vi "get swerve refs.vi"(8 "error in (no error)":errorcluster) -> (0 "error out":errorcluster, 2 "Swerve refs":cluster{"Driver":T1, "Steer":T1, "Encoder":T6}[](array[cluster]))   [LabVIEW 2023]
uses:
  <vilib>/Rock Robotics/WPI/MotorControl/WPI_MotorControlDeviceRef.ctl
  <vilib>/Rock Robotics/WPI/MotorControl/WPI_MotorControlType.ctl
  <vilib>/Rock Robotics/SystemInterfaces/DIO/FPGA_DIOPWMChannel.ctl
  <vilib>/Rock Robotics/WPI/PWM/WPI_PWMDeadband.ctl
  <vilib>/Rock Robotics/SystemInterfaces/DIO/FPGA_DIOChannel.ctl
  <vilib>/Rock Robotics/WPI/ThirdParty/Phoenix-LabVIEW/CANCoder/Controls/CTRE_Phoenix_CANcoder_DeviceRef.ctl
  Global INIT.vi
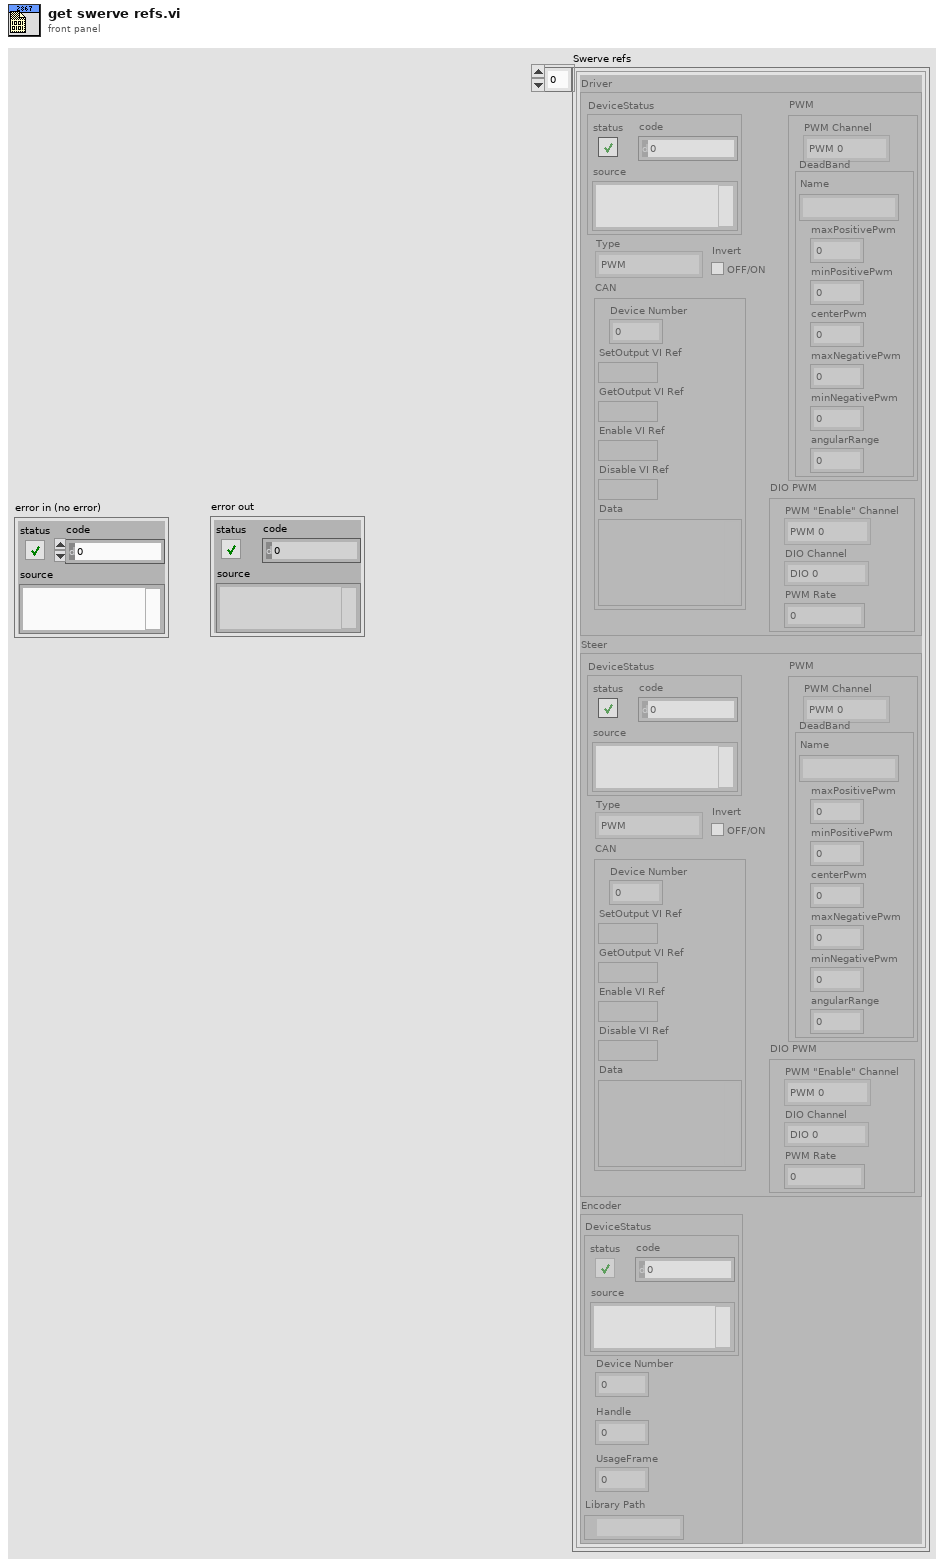
[diagram p1: front panel]
types:
  T1 = typedef "WPI_MotorControlDeviceRef.ctl" = cluster{"DeviceStatus":errorcluster, "Type":T2, "PWM":cluster{"PWM Channel":T3, "DeadBand":T4}, "CAN":cluster{"Device Number":u8, "SetOutput VI Ref":variant, "GetOutput VI Ref":variant, "Enable VI Ref":variant, "Disable VI Ref":variant, "Data":variant}, "Invert":bool, "DIO PWM":cluster{"PWM \"Enable\" Channel":T3, "DIOChannel":T5, "PWM Rate":dbl}}
  T2 = typedef "WPI_MotorControlType.ctl" = enum16{"PWM", "CAN", "DIO PWM"}
  T3 = typedef "FPGA_DIOPWMChannel.ctl" = enum8{"PWM 0", "PWM 1", "PWM 2", "PWM 3", "PWM 4", "PWM 5", "PWM 6", "PWM 7", "PWM 8", "PWM 9", "PWM MXP 0", "PWM MXP 1", "PWM MXP 2", "PWM MXP 3", "PWM MXP 4", "PWM MXP 5", "PWM MXP 6", "PWM MXP 7", "PWM MXP 8", "PWM MXP 9", "Invalid"}
  T4 = typedef "WPI_PWMDeadband.ctl" = cluster{"Name":string, "maxPositivePwm":i32, "minPositivePwm":i32, "centerPwm":i32, "maxNegativePwm":i32, "minNegativePwm":i32, "angularRange":u16}
  T5 = typedef "FPGA_DIOChannel.ctl" = enum8{"DIO 0", "DIO 1", "DIO 2", "DIO 3", "DIO 4", "DIO 5", "DIO 6", "DIO 7", "DIO 8", "DIO 9", "DIO MXP 0", "DIO MXP 1", "DIO MXP 2", "DIO MXP 3", "DIO MXP 4", "DIO MXP 5", "DIO MXP 6", "DIO MXP 7", "DIO MXP 8", "DIO MXP 9", "DIO MXP 10", "DIO MXP 11", "DIO MXP 12", "DIO MXP 13", "DIO MXP 14", "DIO MXP 15", "SPI Port CS1", "SPI Port CS2", "SPI Port CS3", "SPI Port MISO", "SPI Port MOSI", "Invalid"}
  T6 = typedef "CTRE_Phoenix_CANcoder_DeviceRef.ctl" = cluster{"DeviceStatus":errorcluster, "Device Number":u8, "Handle":u64, "UsageFrame":u32, "Library Path":path}
  T7 = typedef "ctrl swerve motor.ctl" = cluster{"description":string, "Installed?":bool, "CAN ID":u8, "refnum name":string, "Invert":bool, "Idle Mode":T8, "Current limiting":T9}
  T8 = typedef "Spark MAX Idle Mode.ctl" = enum16{"Coast", "Brake"}
  T9 = typedef "ctrl Spark MAX current limiting.ctl" = cluster{"Linearized Limit Enabled (F)":bool, "Free Speed Current Limit (20A)":dbl, "Primay Current Limit (80A)":dbl, "Linear Limit RPM (0)":u32}
  T10 = typedef "ctrl CANcoder.ctl" = cluster{"description":string, "Installed?":bool, "CAN ID":u8, "CAN Bus":string, "refnum name":string, "Sensor Direction":bool, "Magnet Offset (Degrees)":dbl}
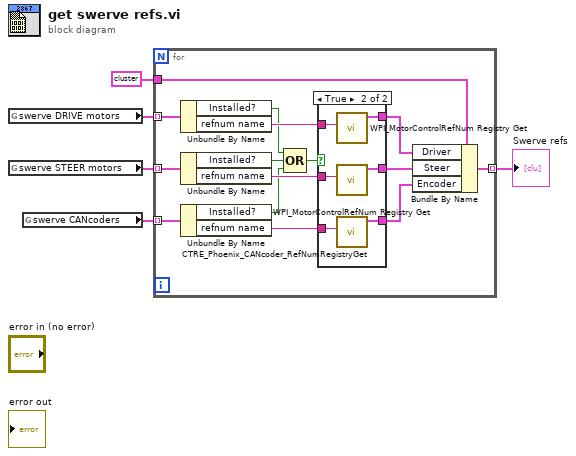
[diagram p0: block diagram]
diagram:
  n1 = global read "Global INIT.vi" "swerve DRIVE motors"() -> (w5:T7[])
  n2 = global read "Global INIT.vi" "swerve STEER motors"() -> (w4:T7[])
  n3 = global read "Global INIT.vi" "swerve CANcoders"() -> (w3:T10[])
  n4 = for {
    tunnel: w5 -> [w20] mode=indexing
    tunnel: w4 -> [w19] mode=indexing
    tunnel: w3 -> [w18] mode=indexing
    tunnel: cluster{"Driver":T1, "Steer":T1, "Encoder":T6} {"Driver"={"DeviceStatus"={"status"=FALSE, "code"=0, "source"=""}, "Type"=enum."PWM", "PWM"={"PWM Channel"=enum."Invalid", "DeadBand"={"Name"="", "maxPositivePwm"=0, "minPositivePwm"=0, "centerPwm"=0, "maxNegativePwm"=0, "minNegativePwm"=0, "angularRange"=0}}, "CAN"={"Device Number"=0, "SetOutput VI Ref"=variant(refnum<vi> refnum), "GetOutput VI Ref"=variant(refnum<vi> refnum), "Enable VI Ref"=variant(refnum<vi> refnum), "Disable VI Ref"=variant(refnum<vi> refnum), "Data"=variant}, "Invert"=FALSE, "DIO PWM"={"PWM \"Enable\" Channel"=enum."Invalid", "DIOChannel"=enum."Invalid", "PWM Rate"=0.0}}, "Steer"={"DeviceStatus"={"status"=FALSE, "code"=0, "source"=""}, "Type"=enum."PWM", "PWM"={"PWM Channel"=enum."Invalid", "DeadBand"={"Name"="", "maxPositivePwm"=0, "minPositivePwm"=0, "centerPwm"=0, "maxNegativePwm"=0, "minNegativePwm"=0, "angularRange"=0}}, "CAN"={"Device Number"=0, "SetOutput VI Ref"=variant(refnum<vi> refnum), "GetOutput VI Ref"=variant(refnum<vi> refnum), "Enable VI Ref"=variant(refnum<vi> refnum), "Disable VI Ref"=variant(refnum<vi> refnum), "Data"=variant}, "Invert"=FALSE, "DIO PWM"={"PWM \"Enable\" Channel"=enum."Invalid", "DIOChannel"=enum."Invalid", "PWM Rate"=0.0}}, "Encoder"={"DeviceStatus"={"status"=FALSE, "code"=0, "source"=""}, "Device Number"=0, "Handle"=0, "UsageFrame"=0, "Library Path"=path ""}} -> [w14]
    tunnel: [w6] -> w1 mode=indexing
    n5 = Unbundle By Name(w20) -> ("Installed?"=w10:bool, "refnum name"=w17:string)
    n6 = Unbundle By Name(w19) -> ("Installed?"=w8:bool, "refnum name"=w16:string)
    n7 = Unbundle By Name(w18) -> ("Installed?"=w9:bool, "refnum name"=w15:string)
    n8 = Compound Arithmetic op=OR(w10, w8, w9) -> (w7:bool)
    n9 = case shown="True" w7 {
      tunnel: w17 -> [_ w26]
      tunnel: w16 -> [_ w25]
      tunnel: w15 -> [_ w24]
      tunnel: [_ w23] -> w13
      tunnel: [_ w22] -> w12
      tunnel: [_ w21] -> w11
      frame False {
      }
      frame True {
        n10 = call <vilib>:"WPI_MotorControlRefNum Registry Get.vi"("refnum name"=w26) -> ("MotorControlDevRef"=w23:T1)  [unwired: 9 in, 1 out]
        n11 = call <vilib>:"WPI_MotorControlRefNum Registry Get.vi"("refnum name"=w25) -> ("MotorControlDevRef"=w22:T1)  [unwired: 9 in, 1 out]
        n12 = call <vilib>:"CTRE_Phoenix_CANcoder_RefNumRegistryGet.vi"("refnum name"=w24) -> ("CTRE_CANcoder_DeviceRef"=w21:T6)  [unwired: 9 in, 1 out]
      }
    }
    n13 = Bundle By Name(cluster=w14, "Driver"=w13, "Steer"=w12, "Encoder"=w11) -> (w6:cluster{"Driver":T1, "Steer":T1, "Encoder":T6})
  }
  "Swerve refs" <- w1
